vi "Reference Queue (Array).vi"(6 "Priority Message? (F)":bool[](array[boolean]), 8 "error in (no error)":errorcluster, 9 "timeout in ms (-1)":i32=-1, 10 "Message Data":variant[](array[variant]), 11 "Tasks":T1[](array[typedef])) -> (0 "error out":errorcluster)   [LabVIEW 2019, in "Task Manager.lvlib"]
doc: "Function to enqueue a Message in a Queue of other Module."
uses:
  Task Manager.lvlib
  State Name.ctl
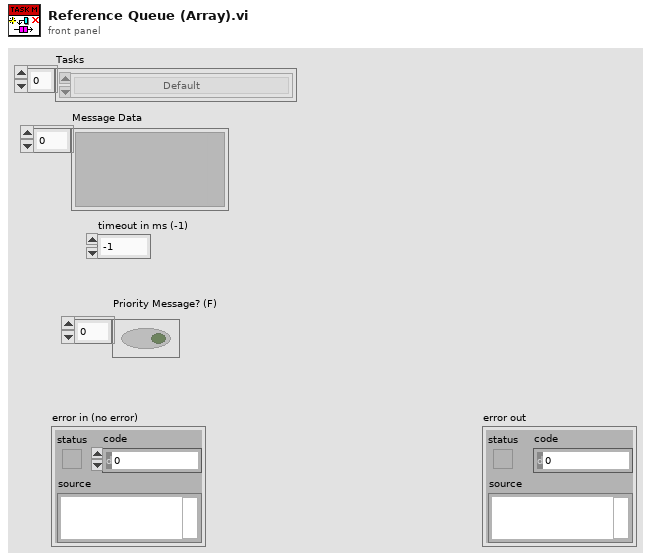
[diagram p1: front panel]
types:
  T1 = typedef "Task Manager.lvlib/State Name.ctl" = enum16{"Default", "Initialize", "Re-Initialize", "Initialize Data", "Initialize Panel", "[Event Structure] Update Data", "Error", "Exit"}
  T2 = typedef "Task Manager.lvlib/Queue Refs.ctl" = refnum<queue>
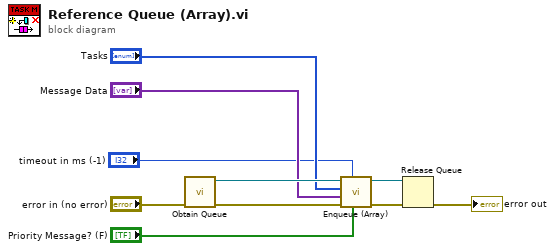
[diagram p0: block diagram]
diagram:
  n1 = call "Obtain Queue.vi"("error in (no error)"="error in (no error)") -> ("error out"=w6:errorcluster, "Message out"=w8:T2)  [unwired: 9 in]
  n2 = call "Enqueue (Array).vi"("Priority Message? Array"="Priority Message? (F)", "timeout in ms (-1)"="timeout in ms (-1)", "error in (no error)"=w6, "Message Data Array"="Message Data", "States"="Tasks", "Message Queue"=w8) -> ("error out"=w2:errorcluster, "Message Queue dub"=w3:T2)  [unwired: 4 in]
  n3 = Release Queue(queue=w3, error in (no error)=w2) -> (error out=→"error out":errorcluster)  [unwired: 1 in, 2 out]
